vi "Folder.vi"(1 "Parameters":T1, 2 "Number of Samples":i32) -> (0 "Folder":dbl[](array[numeric]))   [LabVIEW 2017]
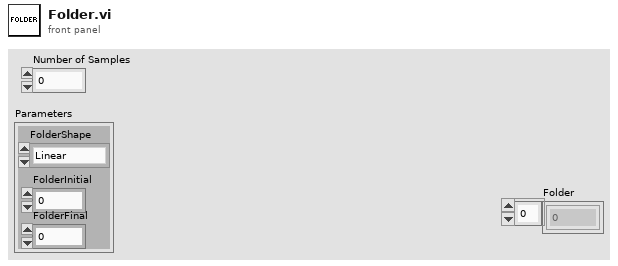
[diagram p1: front panel]
types:
  T1 = cluster{"FolderShape":enum16{"Linear", "Exponential"}, "FolderInitial":dbl, "FolderFinal":dbl}
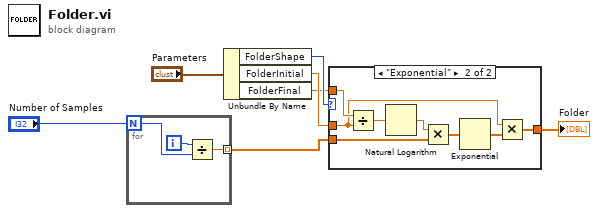
[diagram p0: block diagram]
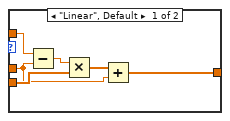
[diagram p2: hidden frame]
diagram:
  n1 = for {
    N: "Number of Samples" -> [w9]
    tunnel: [w8] -> w3 mode=indexing
    i -> [w10]
    n2 = Divide(x=w10, y=w9) -> (x/y=w8:dbl)
  }
  n3 = Unbundle By Name("Parameters") -> ("FolderShape"=w5:enum16{"Linear", "Exponential"}, "FolderInitial"=w2:dbl, "FolderFinal"=w1:dbl)
  n4 = case shown="\"Exponential\"" w5 {
    tunnel: [w15 w20] -> w4
    tunnel: w3 -> [w14 w24]
    tunnel: w2 -> [w12 w18]
    tunnel: w1 -> [w13 w19]
    frame "Linear", Default {
      n5 = Subtract(x=w13, y=w12) -> (x-y=w11:dbl)
      n6 = Multiply(x=w11, y=w14) -> (x*y=w16:dbl[])
      n7 = Add(x=w16, y=w12) -> (x+y=w15:dbl[])
    }
    frame "Exponential" {
      n8 = Divide(x=w19, y=w18) -> (x/y=w17:dbl)
      n9 = Natural Logarithm(1:w17) -> (0:w23:dbl)
      n10 = Multiply(x=w23, y=w24) -> (x*y=w22:dbl[])
      n11 = Exponential(1:w22) -> (0:w21:dbl[])
      n12 = Multiply(x=w18, y=w21) -> (x*y=w20:dbl[])
    }
  }
  "Folder" <- w4
